vi "Step Core.vi"(8 "error in (no error)":errorcluster, 11 "Skyworks Spur Test in":refnum<class "Skyworks Spur Test.lvclass">) -> (0 "error out":errorcluster, 3 "Skyworks Spur Test out":refnum<class "Skyworks Spur Test.lvclass">)   [LabVIEW 2018, in "Skyworks Spur Test.lvlib" / "Skyworks Spur Test.lvclass"]
uses:
  Skyworks Spur Test.lvclass
  C:/Sequence Automation/Plugins/Measurement Interface.lvlibp/Measurement Interface.lvclass
  Plugins/Measurement Interface.lvlibp/Private Methods/Measurement Name/Read Measurement Name.vi
  Plugins/Measurement Interface.lvlibp/Measurement Interface.lvclass
  Plugins/TestStand API Tools (TSAT).lvlibp/Step Actions/TSAT Step Actions.lvlib
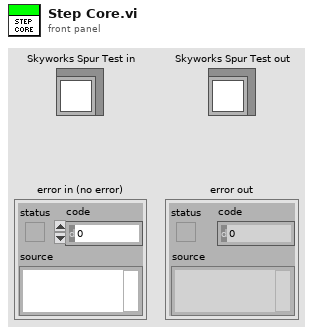
[diagram p1: front panel]
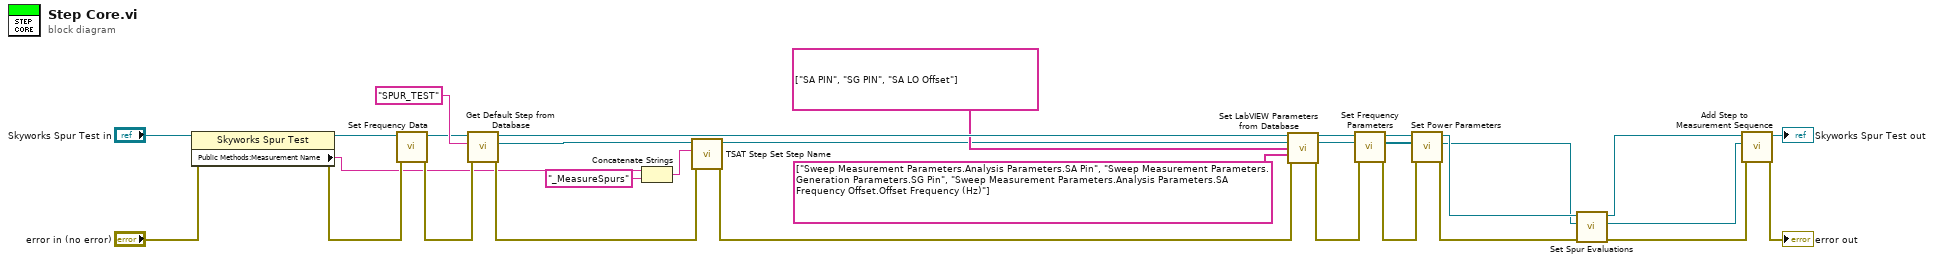
[diagram p0: block diagram]
diagram:
  n1 = property class="Skyworks Spur Test"(reference="Skyworks Spur Test in", error in="error in (no error)") -> (reference out=w15:refnum<class "Skyworks Spur Test.lvclass">, error out=w17:errorcluster, "Public Methods:Measurement Name"=w10:string)
  n2 = call "Set Frequency Data.vi"("error in (no error)"=w17, "Skyworks Spur Test in"=w15) -> ("error out"=w22:errorcluster, "Skyworks Spur Test out"=w21:refnum<class "Skyworks Spur Test.lvclass">)  [unwired: 8 in]
  n3 = call "Get Default Step from Database.vi"("error in (no error)"=w22, "Default Step"="SPUR_TEST", "Measurement Interface in"=w21) -> ("error out"=w28:errorcluster, "Cloned Step"=w13:refnum<k7>, "Measurement Interface out"=w25:refnum<class "Skyworks Spur Test.lvclass">)  [unwired: 6 in]
  n4 = Concatenate Strings(w10, "_MeasureSpurs" ("string")) -> (w11:string)
  n5 = call "TSAT Step Set Step Name.vi"("Error In"=w28, "Name"=w11, "Step In"=w13) -> ("Error Out"=w14:errorcluster, "Step Out"=w12:refnum<k7>)  [unwired: 7 in]
  n6 = call "Set LabVIEW Parameters from Database.vi"("Measurement Interface in"=w25, "Step In"=w12, "Dictionary Keys"=string[] ["SA PIN", "SG PIN", "SA LO Offset"], "LabVIEW Parameter Mapping"=string[] ["Sweep Measurement Parameters.Analysis Parameters.SA Pin", "Sweep Measurement Parameters.Generation Parameters.SG Pin", "Sweep Measurement Parameters.Analysis Parameters.SA Frequency Offset.Offset Frequency (Hz)"], "error in (no error)"=w14) -> ("Measurement Interface out"=w19:refnum<class "Skyworks Spur Test.lvclass">, "Step Out"=w18:refnum<k7>, "error out"=w26:errorcluster)  [unwired: 8 in]
  n7 = call "Set Frequency Parameters.vi"("error in (no error)"=w26, "Step In"=w18, "Skyworks Spur Test in"=w19) -> ("error out"=w20:errorcluster, "Step Out"=w6:refnum<k7>, "Skyworks Spur Test out"=w7:refnum<class "Skyworks Spur Test.lvclass">)  [unwired: 6 in]
  n8 = call "Set Power Parameters.vi"("error in (no error)"=w20, "Step In"=w6, "Skyworks Spur Test in"=w7) -> ("error out"=w8:errorcluster, "Step Out"=w2:refnum<k7>, "Skyworks Spur Test out"=w4:refnum<class "Skyworks Spur Test.lvclass">)  [unwired: 6 in]
  n9 = call "Set Spur Evaluations.vi"("error in (no error)"=w8, "Step In"=w2, "Skyworks Spur Test in"=w4) -> ("error out"=w5:errorcluster, "Step Out"=w1:refnum<k7>, "Skyworks Spur Test out"=w3:refnum<class "Skyworks Spur Test.lvclass">)  [unwired: 6 in]
  n10 = call "Add Step to Measurement Sequence.vi"("error in (no error)"=w5, "Step to Add"=w1, "Measurement Interface in"=w3) -> ("error out"=→"error out":errorcluster, "Measurement Interface out"=→"Skyworks Spur Test out":refnum<class "Skyworks Spur Test.lvclass">)  [unwired: 7 in]
